vi "generate_chirp_3325A.vi"() -> ()   [LabVIEW 2014]
panel:
  in  "GPIB Address":i32=6
  in  "Hz/step":dbl=1.0
  in  "Stop Freq (Hz)":dbl=1000.0
  in  "Start Freq (Hz)":dbl=1.0
  out "Current Freq":dbl format="%#_13g"
  in  "Step Length (s)":i32=1
  in  "Amplitude (V)":dbl=1.0
  in  "Manual Offset (V)":dbl
  in  "Auto Offset":bool=TRUE
  in  "Offset Trim (part per thousand)":i32
  # "VI For Long, Single Chirp with Steady-State to try spinning beads.\nDOES NOT USE CHIRP FUNCTION, JUST SLOWLY CHANGES SINE FREQ"
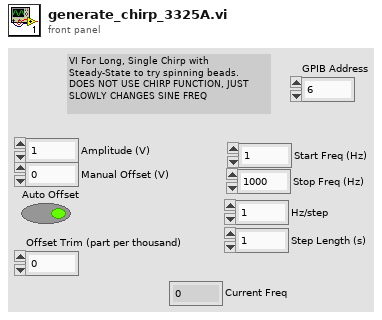
[diagram p1: front panel]
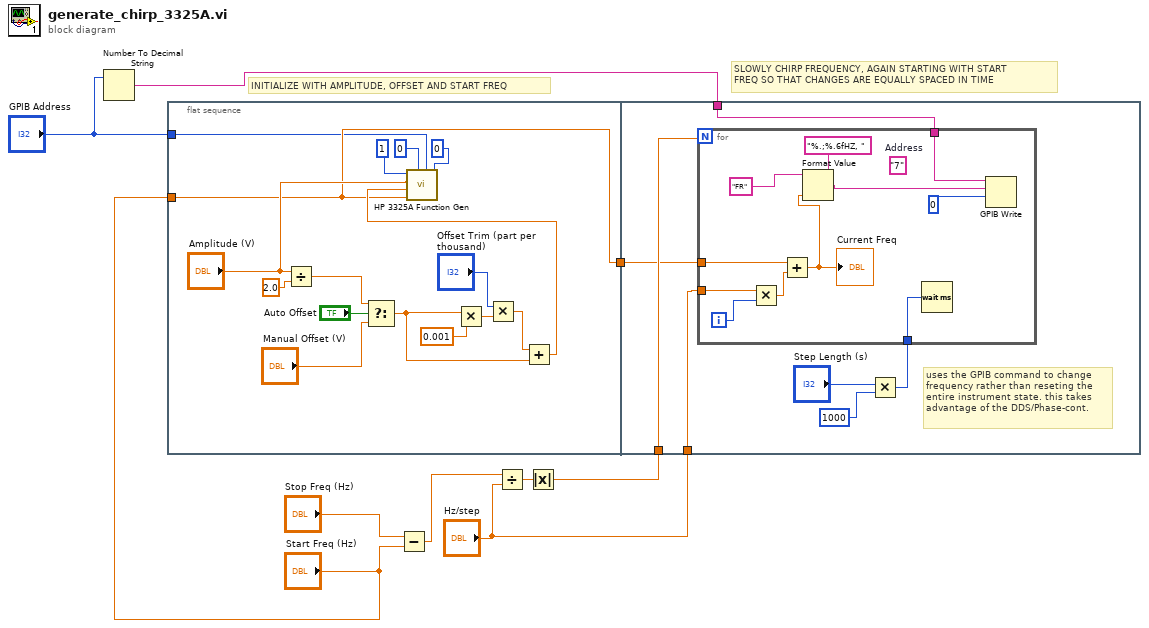
[diagram p0: block diagram]
diagram:
  # "SLOWLY CHIRP FREQUENCY, AGAIN STARTING WITH START\nFREQ SO THAT CHANGES ARE EQUALLY SPACED IN TIME"
  # "INITIALIZE WITH AMPLITUDE, OFFSET AND START FREQ"
  n1 = Number To Decimal String(number="GPIB Address") -> (decimal integer string=w1:string)  [unwired: 1 in]
  n2 = flat-sequence {
    tunnel: "Start Freq (Hz)" -> [w14]
    tunnel: [w14] -> w9
    tunnel: "GPIB Address" -> [w10]
    tunnel: w4 -> [w29]
    tunnel: "Hz/step" -> [w28]
    tunnel: w9 -> [w27]
    tunnel: w1 -> [w26]
    frame #0 {
      n3 = Divide(x="Amplitude (V)", y=2.0) -> (x/y=w23:dbl)
      n4 = Select(t=w23, s="Auto Offset", f="Manual Offset (V)") -> (s? t:f=w21:dbl)
      n5 = Multiply(x=w21, y=0.001) -> (x*y=w18:dbl)
      n6 = Multiply(x="Offset Trim (part per thousand)", y=w18) -> (x*y=w17:dbl)
      n7 = Add(x=w17, y=w21) -> (x+y=w15:dbl)
      n8 = call "HP 3325A Function Gen.vi"("sweep function (none:0)"=0, "GPIB address"=w10, "modulation (off:0)"=0, "frequency (Hz)"=w14, "offset (V)"=w15, "amplitude (V)"="Amplitude (V)", "signal type (dc:0)"=1) -> ()  [unwired: 5 in]
    }
    frame #1 {
      # "uses the GPIB command to change\nfrequency rather than reseting the\nentire instrument state. this takes\nadvantage of the DDS/Phase-cont."
      n9 = Multiply(x="Step Length (s)", y=1000) -> (x*y=w32:i32)
      n10 = for {
        N: w29 -> [_]
        tunnel: w27 -> [w42]
        tunnel: w28 -> [w43]
        tunnel: w32 -> [w39]
        tunnel: w26 -> [w33]
        i -> [w40]
        (unwired) "7"  # Address
        n11 = Multiply(x=w43, y=w40) -> (x*y=w41:dbl)
        n12 = Add(x=w42, y=w41) -> (x+y=w36:dbl)
        "Current Freq" <- w36
        n13 = Format Value(string ("")="FR", format string="%.;%.6fHZ, ", value (0)=w36) -> (output string=w34:string)
        n14 = Wait (ms)(milliseconds to wait=w39) -> ()  [unwired: 1 out]
        n15 = GPIB Write(0:w33, 1:w34, 2:0) -> ()  [unwired: 1 in, 3 out]
      }
    }
  }
  n16 = Subtract(x="Stop Freq (Hz)", y="Start Freq (Hz)") -> (x-y=w7:dbl)
  n17 = Divide(x=w7, y="Hz/step") -> (x/y=w6:dbl)
  n18 = Absolute Value(x=w6) -> (abs(x)=w4:dbl)
